vi "Initialize FPGA Reference.vi"(8 "Error In":errorcluster, 11 "Dashboard In":refnum<class "Dashboard.lvclass">) -> (0 "Error Out":errorcluster, 3 "Dashboard Out":refnum<class "Dashboard.lvclass">)   [LabVIEW 2019, in "Dashboard.lvclass"]
uses:
  Dashboard.lvclass
  <vilib>/FPGAPlugInAG/myRIO-1900/niLvFpga_Open_myRIO-1900.vi
  <vilib>/rvi/interface/common/dynamic/niFpgaDynamicAddResources.vi
  <vilib>/FPGAPlugInAG/Dynamic/niLvFpga_Reset_Dynamic.vi
  Accessors/FPGA Reference/Set FPGA Reference.vi
  Accessors/Processes/Get Processes.vi
  Draw Frame/Accessors/FPGA Reference/Set FPGA Reference.vi
  Audio Analyzer/Accessors/FPGA Reference/Set FPGA Reference.vi
  <vilib>/rvi/interface/nirviOpenFPGA/nirviOpenFPGA.xnode
  Bitfiles/mydashboard_FPGATarget_MainFPGA2_KcnYmAU0WfY.lvbitx
  <vilib>/rvi/interface/nirviMethod/nirviMethod.xnode
  Display Manager/Display Manager.lvclass
  Audio Analyzer/Audio Analyzer.lvclass
  Draw Frame/Draw Frame.lvclass
  Error Handling/Error Handling.lvclass
  Sequencer/Sequencer.lvclass
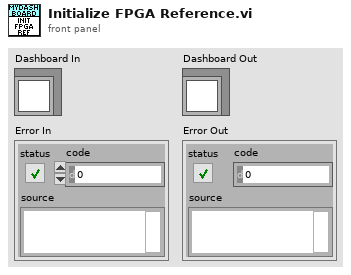
[diagram p1: front panel]
types:
  T1 = typedef "Dashboard.lvclass/Processes.ctl" = cluster{"Display Manager":refnum<class "Display Manager.lvclass">, "Audio Analyzer":refnum<class "Audio Analyzer.lvclass">, "Draw Frame":refnum<class "Draw Frame.lvclass">, "Error Handling":refnum<class "Error Handling.lvclass">, "Sequencer":refnum<class "Sequencer.lvclass">}
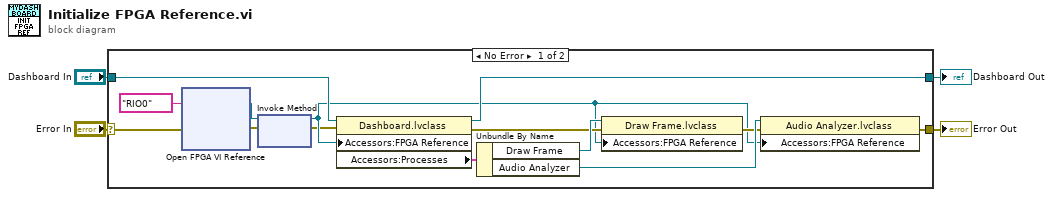
[diagram p0: block diagram]
diagram:
  n1 = case shown="No Error" "Error In" {
    selector: "Error In" -> [w16 w20]
    tunnel: [w9 w20] -> w4
    tunnel: [w18 w19] -> w3
    tunnel: "Dashboard In" -> [w17 w19]
    frame No Error {
      n2 = xnode "Open FPGA VI Reference"("error in"=w16, "resource name"=tag "RIO0") -> ("FPGA VI Reference Out"=w7:refnum<k20>, "error out"=w8:errorcluster)
      n3 = xnode "Invoke Method"("FPGA VI Reference In"=w7, "error in"=w8) -> ("FPGA VI Reference Out"=w6:refnum<k20>, "error out"=w5:errorcluster)
      n4 = property class="Dashboard.lvclass"(reference=w17, error in=w5, "Accessors:FPGA Reference"=w6) -> (reference out=w18:refnum<class "Dashboard.lvclass">, error out=w11:errorcluster, "Accessors:Processes"=w14:T1)
      n5 = Unbundle By Name(w14) -> ("Draw Frame"=w13:refnum<class "Draw Frame.lvclass">, "Audio Analyzer"=w12:refnum<class "Audio Analyzer.lvclass">)
      n6 = property class="Draw Frame.lvclass"(reference=w13, error in=w11, "Accessors:FPGA Reference"=w6) -> (error out=w10:errorcluster)  [unwired: 1 out]
      n7 = property class="Audio Analyzer.lvclass"(reference=w12, error in=w10, "Accessors:FPGA Reference"=w6) -> (error out=w9:errorcluster)  [unwired: 1 out]
    }
    frame Error {
    }
  }
  "Error Out" <- w4
  "Dashboard Out" <- w3
